vi "stage_set_speed.vi"(8 "error in (no error)":errorcluster, 9 "Speed":dbl, 10 "stage name":string, 11 "newport_xps in":refnum<class "newport_xps.lvclass">) -> (0 "error out":errorcluster, 3 "newport_xps out":refnum<class "newport_xps.lvclass">)   [LabVIEW 2015, in "newport_xps.lvclass"]
uses:
  newport_xps.lvclass
  newport_xps.lvclass/newport_xps.ctl
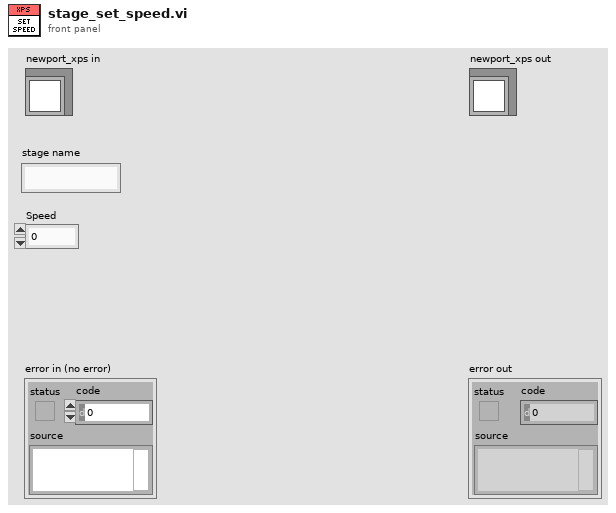
[diagram p1: front panel]
types:
  T1 = cluster{"connection TCP":refnum<k5>, "LogTo File":bool, "Log File refnum":refnum<file>, "no error if error log":bool}
  T2 = cluster{"Velocity (units/seconds)":dbl, "Acceleration (units/seconds²)":dbl, "Minimum Jerk Time (seconds)":dbl, "Maximum Jerk Time (seconds)":dbl}
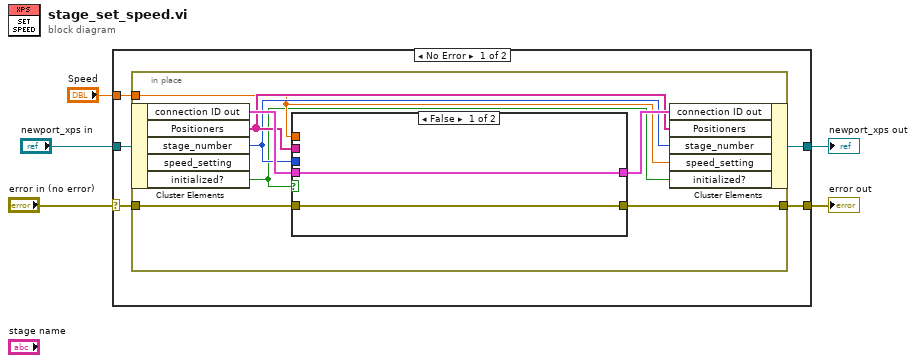
[diagram p0: block diagram]
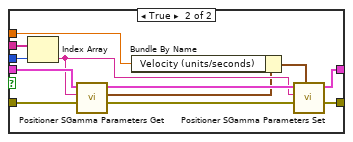
[diagram p2: hidden frame]
diagram:
  n1 = case shown="No Error" "error in (no error)" {
    selector: "error in (no error)" -> [w9 w34]
    tunnel: "newport_xps in" -> [w10 w33]
    tunnel: [w8 w33] -> w2
    tunnel: [w7 w34] -> w3
    tunnel: "Speed" -> [w6 _]
    frame No Error {
      n2 = in-place {
        in-place-border: w9 -> [w17]
        in-place-border: [w15] -> w7
        in-place-border: w6 -> [w12]
        n3 = in-place-cluster #1(w10) -> ("connection ID out"=w16:T1, "Positioners"=w14:string[], "stage_number"=w13:i32, "initialized?"=w11:bool)  [unwired: 1 out]
        n4 = case shown="False" w11 {
          tunnel: [w20 w32] -> w18
          tunnel: w17 -> [w19 w31]
          tunnel: w16 -> [w20 w29]
          tunnel: [w19 w24] -> w15
          tunnel: w14 -> [_ w23]
          tunnel: w13 -> [_ w22]
          tunnel: w12 -> [_ w21]
          frame False {
          }
          frame True {
            n5 = Index Array(array=w23, index=w22) -> (element=w27:string)
            n6 = call "Positioner SGamma Parameters Get.vi"("XPS error in (no error)"=w31, "Positioner Name (250 c max)"=w27, "connection ID in"=w29) -> ("XPS error out"=w30:errorcluster, "SGamma Parameters"=w26:T2, "connection ID out"=w28:T1)  [unwired: 5 in, 1 out]
            n7 = Bundle By Name(cluster=w26, "Velocity (units/seconds)"=w21) -> (w25:T2)
            n8 = call "Positioner SGamma Parameters Set.vi"("SGamma Parameters"=w25, "XPS error in (no error)"=w30, "Positioner Name (250 c max)"=w27, "connection ID in"=w28) -> ("XPS error out"=w24:errorcluster, "connection ID out"=w32:T1)  [unwired: 5 in, 1 out]
          }
        }
        n9 = in-place-cluster #1("connection ID out"=w18, "Positioners"=w14, "stage_number"=w13, "speed_setting"=w12, "initialized?"=w11) -> (w8:refnum<class "newport_xps.lvclass">)
      }
    }
    frame Error {
    }
  }
  "error out" <- w3
  "newport_xps out" <- w2
